vi "Multi Dut Cmd_Header Setting F12_B1.vi"(0 "WS1050/51":bool=TRUE, 5 "Cmin/Act":bool=TRUE, 9 "Test Seq":i32(ring) items=["C1_C2_C3", "C2_C1_C3", "C3_C2_C1", "ALL"], 11 "error in (no error)":errorcluster) -> (1 "Name 1":string[](array[string]), 2 "Name_ALL":string[](array[string]), 3 "Name 2":string[](array[string]), 4 "Name Header":string[](array[string]), 6 "Name 3":string[](array[string]), 10 "Cmd 3":string[](array[string]), 12 "Cmd 1":string[](array[string]), 13 "Extended Cmd":string[](array[string]), 14 "Cmd 2":string[](array[string]), 15 "error out":errorcluster)   [LabVIEW 2012]
panel:
  in  "Cmd 50":string[](array[string])=["00", "01", "00", "02", "00", "04", "00"]
  in  "Name 50":string[](array[string])=["Min", "F1", "F1_OFF", "F2", "F2_OFF", "S1", "S1_OFF"]
  in  "Cmd 51 Cmin":string[](array[string])=["00", "00", "00", "00", "00", "00", "00", "00", "00", "00", "00", "00", "00", "00", "00", "00", "00", "00", "00", "00", "00", "00", "00", "00", "00", "00", "00", "00", "00"]
  in  "Cmd 50 Cmin":string[](array[string])=["00", "00", "00", "00", "00", "00", "00", "00", "00", "00", "00", "00", "00", "00", "00", "00", "00", "00", "00", "00", "00", "00", "00", "00", "00", "00", "00", "00", "00", "00", "00", "00", "00", "00", "00"]
  in  "Cmd 51":string[](array[string])=["00", "01", "00", "02", "00", "04", "00", "08", "04", "0C", "08", "10", "0C", "14", "10", "18", "14", "1C", "18", "20", "1C", "24", "20", "28", "24", "2C", "28", "2F", "00"]
  in  "Name 51":string[](array[string])=["Min", "F1", "F1_OFF", "F2", "F2_OFF", "S1", "S1_OFF", "S2", "S2_OFF", "S3", "S3_OFF", "S4", "S4_OFF", "S5", "S5_OFF", "S6", "S6_OFF", "S7", "S7_OFF", "S8", "S8_OFF", "S9", "S9_OFF", "S10", "S10_OFF", "S11", "S11_OFF", "S11_F12", "Min2"]
  # "Updated to work with Ver1.4:\n\n1.  updated Test Seq by adding a \"ALL\"\nto measure all three banks at the same time"
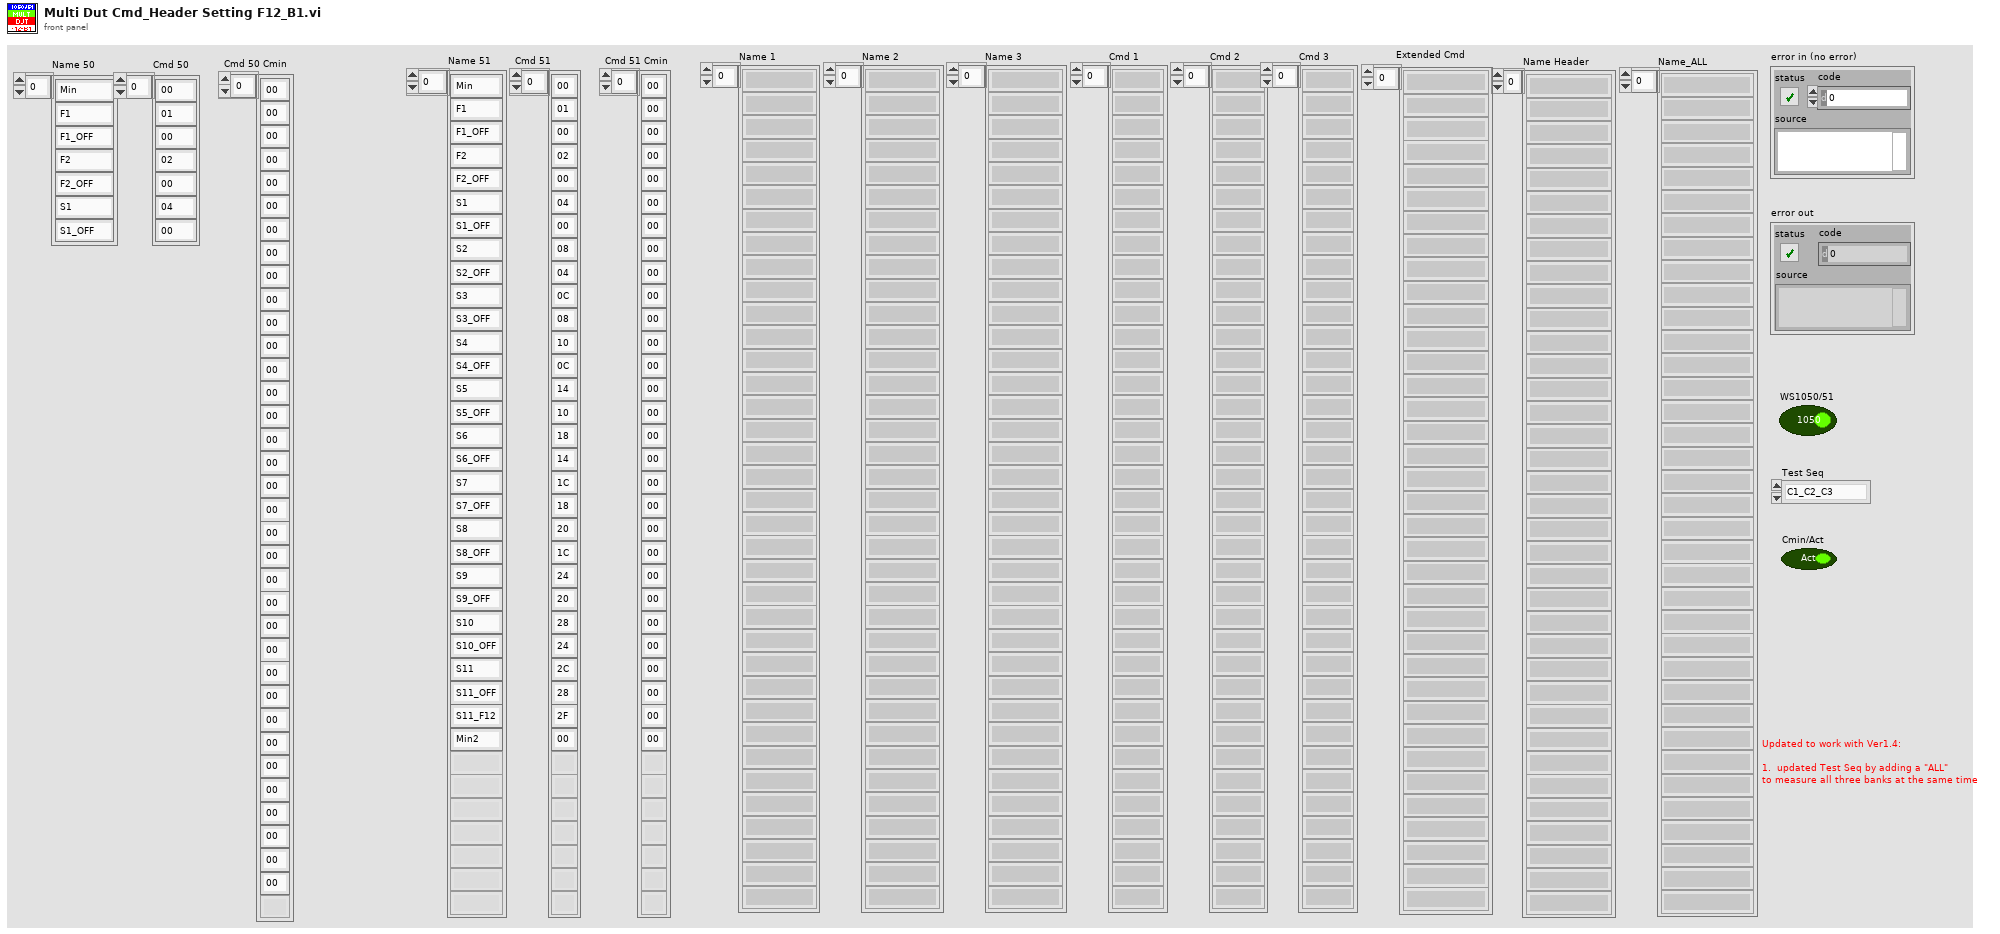
[diagram p1: front panel]
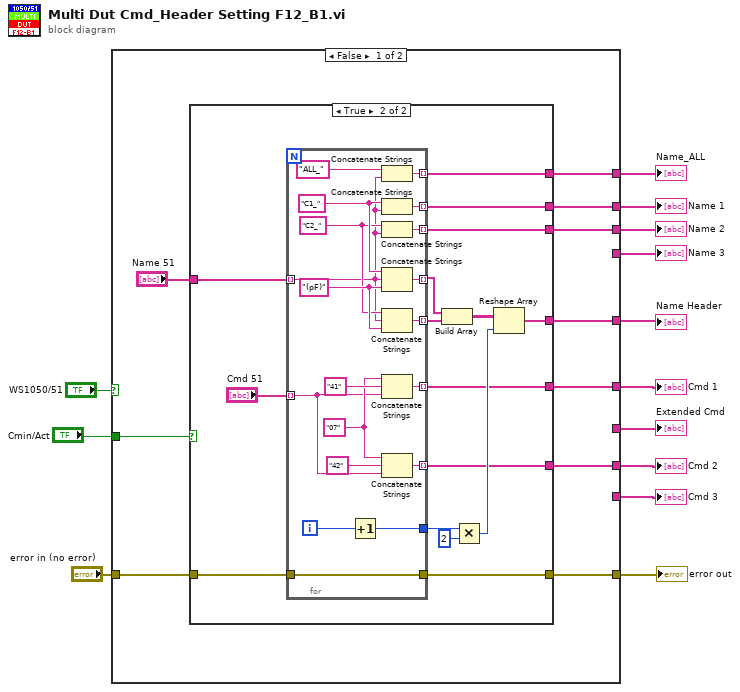
[diagram p0: block diagram]
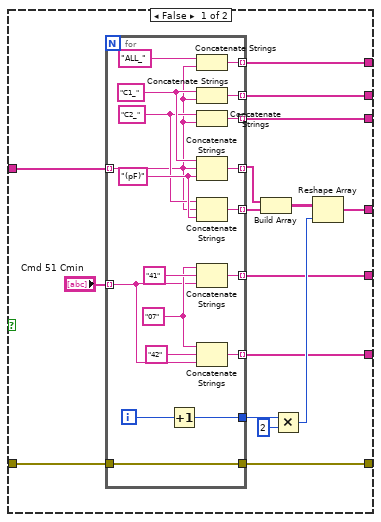
[diagram p2: hidden frame]
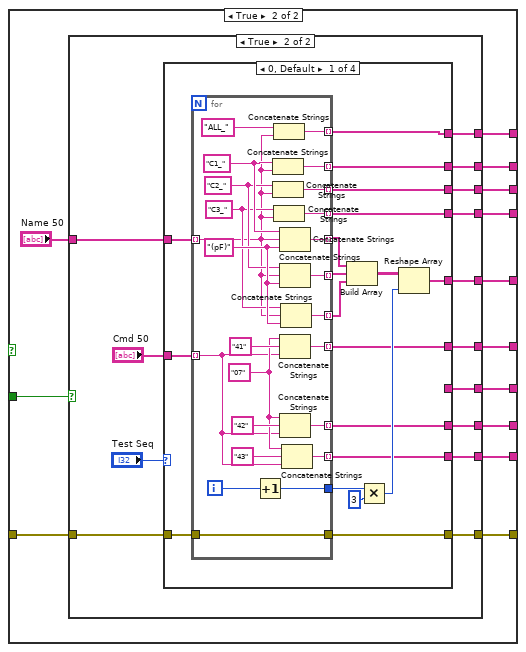
[diagram p3: hidden frame]
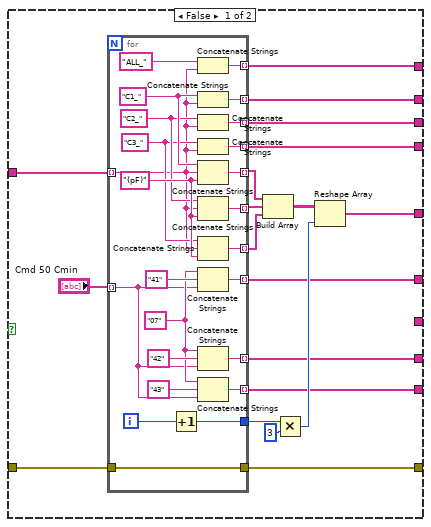
[diagram p4: hidden frame]
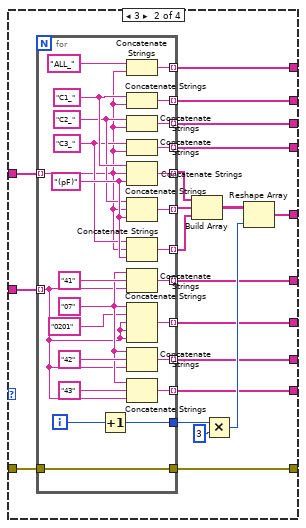
[diagram p5: hidden frame]
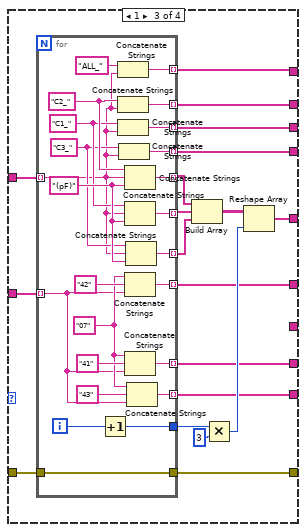
[diagram p6: hidden frame]
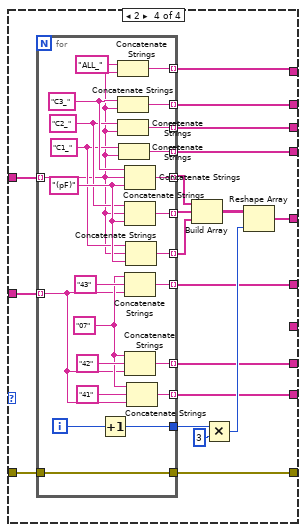
[diagram p7: hidden frame]
diagram:
  n1 = case shown="False" "WS1050/51" {
    tunnel: "error in (no error)" -> [w20 w106]
    tunnel: [w19 w105] -> w12
    tunnel: [w21 w104] -> w10
    tunnel: [w23 w103] -> w9
    tunnel: [w22 w102] -> w8
    tunnel: [_ w101] -> w7
    tunnel: [w18 w100] -> w6
    tunnel: [w17 w99] -> w5
    tunnel: [_ w98] -> w4
    tunnel: "Cmin/Act" -> [w16 w97]
    tunnel: [_ w96] -> w2
    tunnel: [w14 w95] -> w1
    frame False {
      n2 = case shown="True" w16 {
        tunnel: [w32 w68] -> w23
        tunnel: [w31 w67] -> w22
        tunnel: [w30 w66] -> w21
        tunnel: w20 -> [w25 w64]
        tunnel: [w27 w63] -> w19
        tunnel: [w29 w62] -> w18
        tunnel: [w28 w61] -> w17
        tunnel: "Name 51" -> [w26 w60]
        tunnel: [w24 w59] -> w14
        frame False {
          n3 = for {
            tunnel: w26 -> [w42] mode=indexing
            tunnel: [w58] -> w34 mode=indexing
            tunnel: [w57] -> w35 mode=indexing
            tunnel: "Cmd 51 Cmin" -> [w51] mode=indexing
            tunnel: [w55] -> w29 mode=indexing
            tunnel: [w53] -> w28 mode=indexing
            tunnel: [w47] -> w32 mode=indexing
            tunnel: [w49] -> w38
            tunnel: [w46] -> w31 mode=indexing
            tunnel: w25 -> [w43]
            tunnel: [w43] -> w27
            tunnel: [w40] -> w24 mode=indexing
            i -> [w48]
            w44 = "C2_" ("string")
            w50 = "(pF)" ("string")
            w45 = "C1_" ("string")
            w52 = "07" ("string")
            n4 = Increment(x=w48) -> (x+1=w49:i32)
            n5 = Concatenate Strings("ALL_" ("string"), w42) -> (w40:string)
            n6 = Concatenate Strings(w45, w42) -> (w47:string)
            n7 = Concatenate Strings(w44, w42) -> (w46:string)
            n8 = Concatenate Strings(w45, w42, w50) -> (w58:string)
            n9 = Concatenate Strings(w44, w42, w50) -> (w57:string)
            n10 = Concatenate Strings(w52, "41" ("string"), w51) -> (w55:string)
            n11 = Concatenate Strings(w52, "42" ("string"), w51) -> (w53:string)
          }
          n12 = Build Array(w34, w35) -> (w36:string[][])
          n13 = Multiply(x=w38, y=2) -> (x*y=w37:i32)
          n14 = Reshape Array(w36, w37) -> (w30:string[])
        }
        frame True {
          n15 = for {
            tunnel: w60 -> [w77] mode=indexing
            tunnel: [w93] -> w69 mode=indexing
            tunnel: [w92] -> w70 mode=indexing
            tunnel: "Cmd 51" -> [w86] mode=indexing
            tunnel: [w90] -> w62 mode=indexing
            tunnel: [w88] -> w61 mode=indexing
            tunnel: [w78] -> w68 mode=indexing
            tunnel: [w84] -> w73
            tunnel: [w82] -> w67 mode=indexing
            tunnel: w64 -> [w79]
            tunnel: [w79] -> w63
            tunnel: [w75] -> w59 mode=indexing
            i -> [w83]
            w80 = "C2_" ("string")
            w85 = "(pF)" ("string")
            w81 = "C1_" ("string")
            w87 = "07" ("string")
            n16 = Increment(x=w83) -> (x+1=w84:i32)
            n17 = Concatenate Strings("ALL_" ("string"), w77) -> (w75:string)
            n18 = Concatenate Strings(w81, w77) -> (w78:string)
            n19 = Concatenate Strings(w80, w77) -> (w82:string)
            n20 = Concatenate Strings(w81, w77, w85) -> (w93:string)
            n21 = Concatenate Strings(w80, w77, w85) -> (w92:string)
            n22 = Concatenate Strings(w87, "41" ("string"), w86) -> (w90:string)
            n23 = Concatenate Strings(w87, "42" ("string"), w86) -> (w88:string)
          }
          n24 = Build Array(w69, w70) -> (w71:string[][])
          n25 = Multiply(x=w73, y=2) -> (x*y=w72:i32)
          n26 = Reshape Array(w71, w72) -> (w66:string[])
        }
      }
    }
    frame True {
      n27 = case shown="True" w97 {
        tunnel: w106 -> [w110 w163]
        tunnel: [w111 w162] -> w105
        tunnel: [w115 w161] -> w104
        tunnel: [w118 w160] -> w103
        tunnel: [w117 w159] -> w102
        tunnel: [w116 w158] -> w101
        tunnel: [w114 w157] -> w100
        tunnel: [w113 w156] -> w99
        tunnel: [w112 w155] -> w98
        tunnel: "Name 50" -> [w109 w153]
        tunnel: [_ w152] -> w96
        tunnel: [w108 w151] -> w95
        frame False {
          n28 = for {
            tunnel: w109 -> [w128] mode=indexing
            tunnel: [w149] -> w125 mode=indexing
            tunnel: [w148] -> w124 mode=indexing
            tunnel: [w147] -> w123 mode=indexing
            tunnel: "Cmd 50 Cmin" -> [w140] mode=indexing
            tunnel: [w145] -> w114 mode=indexing
            tunnel: [w143] -> w113 mode=indexing
            tunnel: [w139] -> w112 mode=indexing
            tunnel: [w129] -> w118 mode=indexing
            tunnel: [w137] -> w120
            tunnel: [w135] -> w117 mode=indexing
            tunnel: [w134] -> w116 mode=indexing
            tunnel: w110 -> [w130]
            tunnel: [w130] -> w111
            tunnel: [w126] -> w108 mode=indexing
            i -> [w136]
            w131 = "C3_" ("string")
            w132 = "C2_" ("string")
            w138 = "(pF)" ("string")
            w133 = "C1_" ("string")
            w142 = "07" ("string")
            n29 = Increment(x=w136) -> (x+1=w137:i32)
            n30 = Concatenate Strings("ALL_" ("string"), w128) -> (w126:string)
            n31 = Concatenate Strings(w133, w128) -> (w129:string)
            n32 = Concatenate Strings(w132, w128) -> (w135:string)
            n33 = Concatenate Strings(w131, w128) -> (w134:string)
            n34 = Concatenate Strings(w133, w128, w138) -> (w149:string)
            n35 = Concatenate Strings(w132, w128, w138) -> (w148:string)
            n36 = Concatenate Strings(w131, w128, w138) -> (w147:string)
            n37 = Concatenate Strings(w142, "41" ("string"), w140) -> (w145:string)
            n38 = Concatenate Strings(w142, "42" ("string"), w140) -> (w143:string)
            n39 = Concatenate Strings(w142, "43" ("string"), w140) -> (w139:string)
          }
          n40 = Build Array(w125, w124, w123) -> (w122:string[][])
          n41 = Multiply(x=w120, y=3) -> (x*y=w121:i32)
          n42 = Reshape Array(w122, w121) -> (w115:string[])
        }
        frame True {
          n43 = case shown="0, Default" "Test Seq" {
            tunnel: w153 -> [w182 w226 w271 w314]
            tunnel: "Cmd 50" -> [w181 w225 w270 w313]
            tunnel: w163 -> [w173 w217 w262 w305]
            tunnel: [w172 w216 w261 w304] -> w162
            tunnel: [w171 w215 w260 w303] -> w161
            tunnel: [w170 w214 w259 w302] -> w160
            tunnel: [w169 w213 w258 w301] -> w159
            tunnel: [w168 w212 w257 w300] -> w158
            tunnel: [w167 w211 w256 w299] -> w157
            tunnel: [w166 w210 w255 w298] -> w156
            tunnel: [w165 w209 w254 w297] -> w155
            tunnel: [_ w208 _ _] -> w152
            tunnel: [w164 w207 w253 w296] -> w151
            frame 0, Default {
              n44 = for {
                tunnel: w182 -> [w185] mode=indexing
                tunnel: [w206] -> w180 mode=indexing
                tunnel: [w205] -> w179 mode=indexing
                tunnel: [w204] -> w178 mode=indexing
                tunnel: w181 -> [w187] mode=indexing
                tunnel: [w202] -> w167 mode=indexing
                tunnel: [w200] -> w166 mode=indexing
                tunnel: [w198] -> w165 mode=indexing
                tunnel: [w186] -> w170 mode=indexing
                tunnel: [w196] -> w175
                tunnel: [w194] -> w169 mode=indexing
                tunnel: [w193] -> w168 mode=indexing
                tunnel: w173 -> [w189]
                tunnel: [w189] -> w172
                tunnel: [w183] -> w164 mode=indexing
                i -> [w195]
                w190 = "C3_" ("string")
                w191 = "C2_" ("string")
                w197 = "(pF)" ("string")
                w192 = "C1_" ("string")
                w188 = "07" ("string")
                n45 = Increment(x=w195) -> (x+1=w196:i32)
                n46 = Concatenate Strings(w192, w185) -> (w186:string)
                n47 = Concatenate Strings(w191, w185) -> (w194:string)
                n48 = Concatenate Strings("ALL_" ("string"), w185) -> (w183:string)
                n49 = Concatenate Strings(w190, w185) -> (w193:string)
                n50 = Concatenate Strings(w192, w185, w197) -> (w206:string)
                n51 = Concatenate Strings(w191, w185, w197) -> (w205:string)
                n52 = Concatenate Strings(w188, "41" ("string"), w187) -> (w202:string)
                n53 = Concatenate Strings(w188, "42" ("string"), w187) -> (w200:string)
                n54 = Concatenate Strings(w190, w185, w197) -> (w204:string)
                n55 = Concatenate Strings(w188, "43" ("string"), w187) -> (w198:string)
              }
              n56 = Build Array(w180, w179, w178) -> (w177:string[][])
              n57 = Multiply(x=w175, y=3) -> (x*y=w176:i32)
              n58 = Reshape Array(w177, w176) -> (w171:string[])
            }
            frame 3 {
              n59 = for {
                tunnel: w226 -> [w229] mode=indexing
                tunnel: [w252] -> w224 mode=indexing
                tunnel: [w251] -> w223 mode=indexing
                tunnel: [w250] -> w222 mode=indexing
                tunnel: w225 -> [w231] mode=indexing
                tunnel: [w248] -> w211 mode=indexing
                tunnel: [w246] -> w210 mode=indexing
                tunnel: [w244] -> w209 mode=indexing
                tunnel: [w240] -> w214 mode=indexing
                tunnel: [w242] -> w219
                tunnel: [w239] -> w213 mode=indexing
                tunnel: [w238] -> w212 mode=indexing
                tunnel: w217 -> [w234]
                tunnel: [w234] -> w216
                tunnel: [w230] -> w208 mode=indexing
                tunnel: [w227] -> w207 mode=indexing
                i -> [w241]
                w235 = "C3_" ("string")
                w236 = "C2_" ("string")
                w243 = "(pF)" ("string")
                w237 = "C1_" ("string")
                w233 = "07" ("string")
                n60 = Increment(x=w241) -> (x+1=w242:i32)
                n61 = Concatenate Strings("ALL_" ("string"), w229) -> (w227:string)
                n62 = Concatenate Strings(w237, w229) -> (w240:string)
                n63 = Concatenate Strings(w236, w229) -> (w239:string)
                n64 = Concatenate Strings(w235, w229) -> (w238:string)
                n65 = Concatenate Strings(w237, w229, w243) -> (w252:string)
                n66 = Concatenate Strings(w236, w229, w243) -> (w251:string)
                n67 = Concatenate Strings(w235, w229, w243) -> (w250:string)
                n68 = Concatenate Strings(w233, "41" ("string"), w231) -> (w248:string)
                n69 = Concatenate Strings(w233, "0201" ("string"), w231, w231, w231) -> (w230:string)
                n70 = Concatenate Strings(w233, "42" ("string"), w231) -> (w246:string)
                n71 = Concatenate Strings(w233, "43" ("string"), w231) -> (w244:string)
              }
              n72 = Build Array(w224, w223, w222) -> (w221:string[][])
              n73 = Multiply(x=w219, y=3) -> (x*y=w220:i32)
              n74 = Reshape Array(w221, w220) -> (w215:string[])
            }
            frame 1 {
              n75 = for {
                tunnel: w271 -> [w274] mode=indexing
                tunnel: [w295] -> w269 mode=indexing
                tunnel: [w294] -> w268 mode=indexing
                tunnel: [w293] -> w267 mode=indexing
                tunnel: w270 -> [w286] mode=indexing
                tunnel: [w291] -> w256 mode=indexing
                tunnel: [w289] -> w255 mode=indexing
                tunnel: [w285] -> w254 mode=indexing
                tunnel: [w281] -> w259 mode=indexing
                tunnel: [w283] -> w264
                tunnel: [w280] -> w258 mode=indexing
                tunnel: [w279] -> w257 mode=indexing
                tunnel: w262 -> [w275]
                tunnel: [w275] -> w261
                tunnel: [w272] -> w253 mode=indexing
                i -> [w282]
                w276 = "C3_" ("string")
                w277 = "C1_" ("string")
                w284 = "(pF)" ("string")
                w278 = "C2_" ("string")
                w288 = "07" ("string")
                n76 = Increment(x=w282) -> (x+1=w283:i32)
                n77 = Concatenate Strings("ALL_" ("string"), w274) -> (w272:string)
                n78 = Concatenate Strings(w278, w274) -> (w281:string)
                n79 = Concatenate Strings(w277, w274) -> (w280:string)
                n80 = Concatenate Strings(w276, w274) -> (w279:string)
                n81 = Concatenate Strings(w278, w274, w284) -> (w295:string)
                n82 = Concatenate Strings(w277, w274, w284) -> (w294:string)
                n83 = Concatenate Strings(w288, "42" ("string"), w286) -> (w291:string)
                n84 = Concatenate Strings(w288, "41" ("string"), w286) -> (w289:string)
                n85 = Concatenate Strings(w276, w274, w284) -> (w293:string)
                n86 = Concatenate Strings(w288, "43" ("string"), w286) -> (w285:string)
              }
              n87 = Build Array(w269, w268, w267) -> (w266:string[][])
              n88 = Multiply(x=w264, y=3) -> (x*y=w265:i32)
              n89 = Reshape Array(w266, w265) -> (w260:string[])
            }
            frame 2 {
              n90 = for {
                tunnel: w314 -> [w317] mode=indexing
                tunnel: [w338] -> w312 mode=indexing
                tunnel: [w337] -> w311 mode=indexing
                tunnel: [w336] -> w310 mode=indexing
                tunnel: w313 -> [w329] mode=indexing
                tunnel: [w334] -> w299 mode=indexing
                tunnel: [w332] -> w298 mode=indexing
                tunnel: [w328] -> w297 mode=indexing
                tunnel: [w324] -> w302 mode=indexing
                tunnel: [w326] -> w307
                tunnel: [w323] -> w301 mode=indexing
                tunnel: [w322] -> w300 mode=indexing
                tunnel: w305 -> [w318]
                tunnel: [w318] -> w304
                tunnel: [w315] -> w296 mode=indexing
                i -> [w325]
                w319 = "C1_" ("string")
                w320 = "C2_" ("string")
                w327 = "(pF)" ("string")
                w321 = "C3_" ("string")
                w331 = "07" ("string")
                n91 = Increment(x=w325) -> (x+1=w326:i32)
                n92 = Concatenate Strings("ALL_" ("string"), w317) -> (w315:string)
                n93 = Concatenate Strings(w321, w317) -> (w324:string)
                n94 = Concatenate Strings(w320, w317) -> (w323:string)
                n95 = Concatenate Strings(w319, w317) -> (w322:string)
                n96 = Concatenate Strings(w321, w317, w327) -> (w338:string)
                n97 = Concatenate Strings(w320, w317, w327) -> (w337:string)
                n98 = Concatenate Strings(w331, "43" ("string"), w329) -> (w334:string)
                n99 = Concatenate Strings(w331, "42" ("string"), w329) -> (w332:string)
                n100 = Concatenate Strings(w319, w317, w327) -> (w336:string)
                n101 = Concatenate Strings(w331, "41" ("string"), w329) -> (w328:string)
              }
              n102 = Build Array(w312, w311, w310) -> (w309:string[][])
              n103 = Multiply(x=w307, y=3) -> (x*y=w308:i32)
              n104 = Reshape Array(w309, w308) -> (w303:string[])
            }
          }
        }
      }
    }
  }
  "error out" <- w12
  "Name Header" <- w10
  "Name 1" <- w9
  "Name 2" <- w8
  "Name 3" <- w7
  "Cmd 1" <- w6
  "Cmd 2" <- w5
  "Cmd 3" <- w4
  "Extended Cmd" <- w2
  "Name_ALL" <- w1
